vi "Write Boolean Notifier.vi"(8 "error in (no error)":errorcluster, 10 "Boolean Notifier":refnum<notifier>, 11 "Example Source in":refnum<class "Example Source.lvclass">) -> (0 "error out":errorcluster, 3 "Example Source out":refnum<class "Example Source.lvclass">)   [LabVIEW 2016, in "Example Source.lvlib" / "Example Source.lvclass"]
uses:
  Example Source.lvclass
  Example Source.lvclass/Example Source.ctl
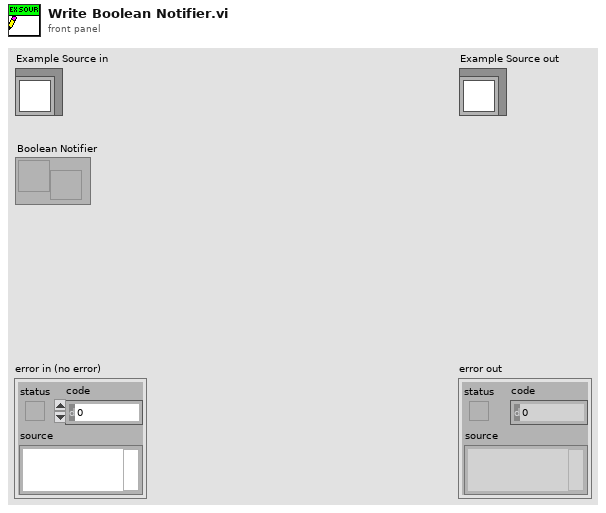
[diagram p1: front panel]
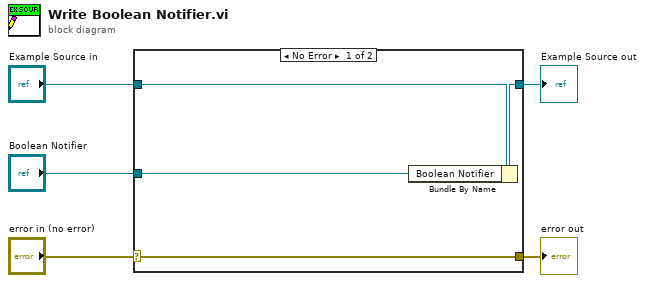
[diagram p0: block diagram]
diagram:
  n1 = case shown="No Error" "error in (no error)" {
    selector: "error in (no error)" -> [w9 w10]
    tunnel: [w9 w10] -> w4
    tunnel: [w7 w11] -> w2
    tunnel: "Example Source in" -> [w8 w11]
    tunnel: "Boolean Notifier" -> [w6 _]
    frame No Error {
      n2 = Bundle By Name(cluster=w8, "Boolean Notifier"=w6) -> (w7:refnum<class "Example Source.lvclass">)
    }
    frame Error {
    }
  }
  "error out" <- w4
  "Example Source out" <- w2
